vi "FloodDir.vi"(9 "Intended Dir":T1, 11 "View":i32[](array[numeric])) -> (1 "Free space?":bool=TRUE, 3 "Direction":T1)   [LabVIEW 2020, in "Atom.lvclass"]
uses:
  Atom.lvclass
  Type Defs/Direction Enum.ctl
  Type Defs/SB Type Defs.lvlib
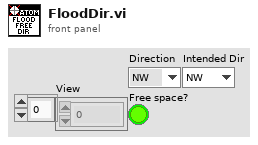
[diagram p1: front panel]
types:
  T1 = typedef "SB Type Defs.lvlib/Direction Enum.ctl" = enum16{"NW", "N", "NE", "E", "SE", "S", "SW", "W"}
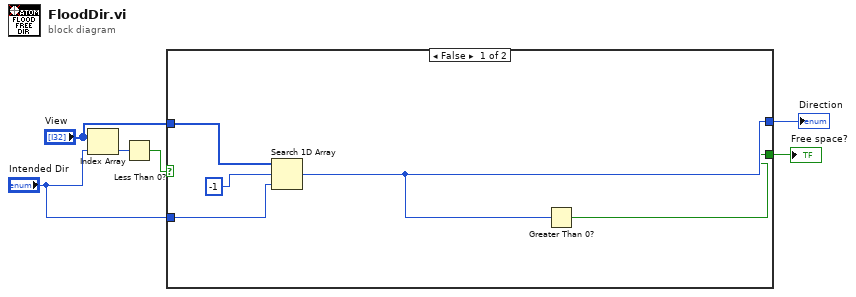
[diagram p0: block diagram]
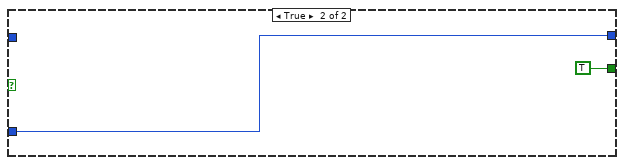
[diagram p2: hidden frame]
diagram:
  n1 = Index Array(array="View", index="Intended Dir") -> (element=w2:i32)
  n2 = Less Than 0?(x=w2) -> (x < 0?=w3:bool)
  n3 = case shown="False" w3 {
    tunnel: [w8 w13] -> w6
    tunnel: [w7 TRUE] -> w5
    tunnel: "View" -> [w11 _]
    tunnel: "Intended Dir" -> [w9 w13]
    frame False {
      n4 = Search 1D Array(1D array=w11, element=-1, start index (0)=w9) -> (index of element=w8:i32)
      n5 = Greater Than 0?(x=w8) -> (x > 0?=w7:bool)
    }
    frame True {
    }
  }
  "Direction" <- w6
  "Free space?" <- w5
